vi "TouchPanel.ReadFKeys.vi"(7 "forced read (F)":bool, 8 "error in (no error)":errorcluster, 9 "Keyset to read":T1[](array[typedef]), 10 "key?":T1, 11 "mode (read key)":T2=enum."read key") -> (0 "error out":errorcluster, 2 "keyPressed":bool, 3 "Keyset out":T1[](array[typedef]))   [LabVIEW 2010]
uses:
  TouchPanel.keyMode.ctl
  TouchPanel.functionKeys.ctl
  LvSecure.dll
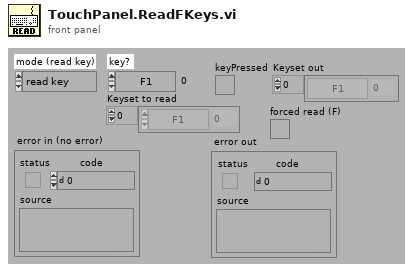
[diagram p1: front panel]
types:
  T1 = typedef "TouchPanel.functionKeys.ctl" = enum32{"F1", "F2", "F3", "F4", "F5", "F6", "F7", "F8", "F9", "F10", "F11", "F12", "Alt F1", "Alt F2", "Alt F3", "Alt F4", "Alt F5", "Alt F6", "Alt F7", "Alt F8", "Alt F9", "Alt F10", "Alt F11", "Alt F12", "Ctrl F1", "Ctrl F2", "Ctrl F3", "Ctrl F4", "Ctrl F5", "Ctrl F6", "Ctrl F7", "Ctrl F8", "Ctrl F9", "Ctrl F10", "Ctrl F11", "Ctrl F12", "Shift F1", "Shift F2", "Shift F3", "Shift F4", "Shift F5", "Shift F6", "Shift F7", "Shift F8", "Shift F9", "Shift F10", "Shift F11", "Shift F12", "Ctrl-Shift", "a", "b", "c", "d", "e", "f", "g", "h", "i", "j", "k", "l", "m", "n", "o", "p", "q", "r", "s", "t", "u", "v", "w", "x", "y", "z", "A", "B", "C", "D", "E", "F", "G", "H", "I", "J", "K", "L", "M", "N", "O", "P", "Q", "R", "S", "T", "U", "V", "W", "X", "Y", "Z", "0", "1", "2", "3", "4", "5", "6", "7", "8", "9", "Left", "Up", "Right", "Down", "Ctrl X", "Backspace", "Tab", "Enter", "Space", "End", "Home", "Insert", "Delete", ".", ","}
  T2 = typedef "TouchPanel.keyMode.ctl" = enum16{"init hook", "update keys", "read key", "read keyset", "read all", "simulate key", "mask keys", "unmask keys", "clear keys", "close hook"}
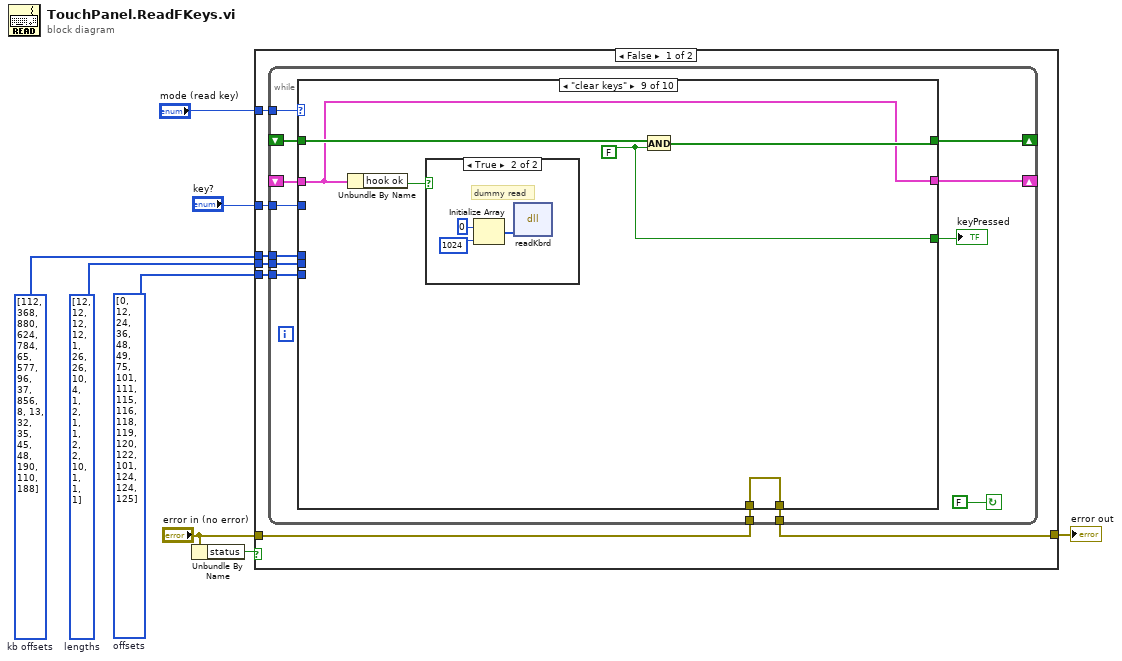
[diagram p0: block diagram]
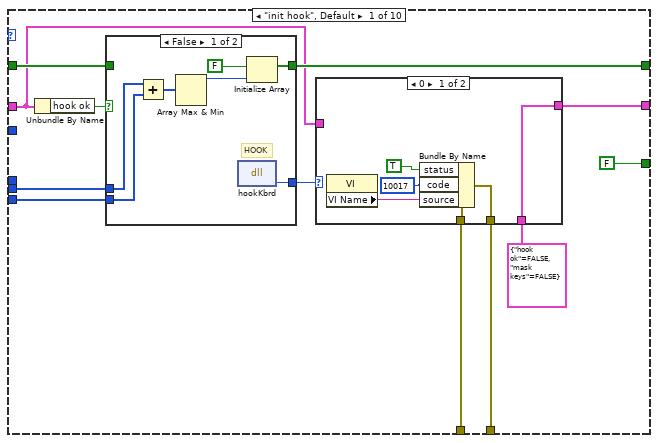
[diagram p2: hidden frame]
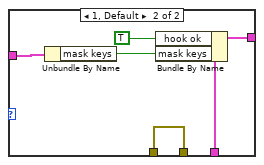
[diagram p3: hidden frame]
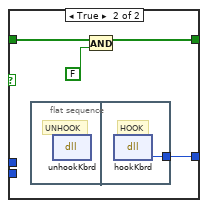
[diagram p4: hidden frame]
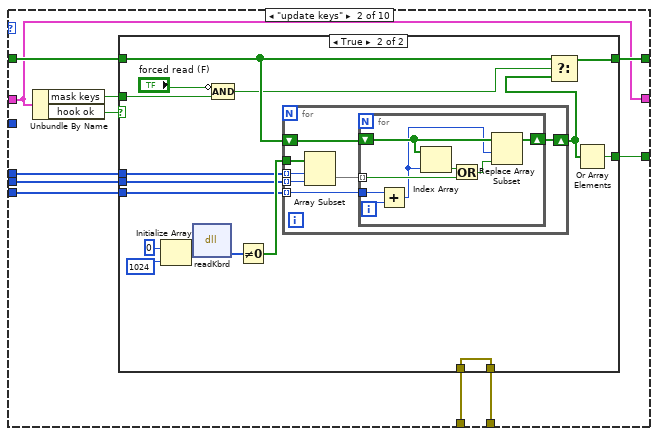
[diagram p5: hidden frame]
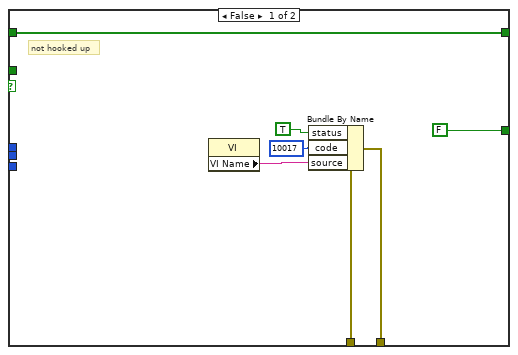
[diagram p6: hidden frame]
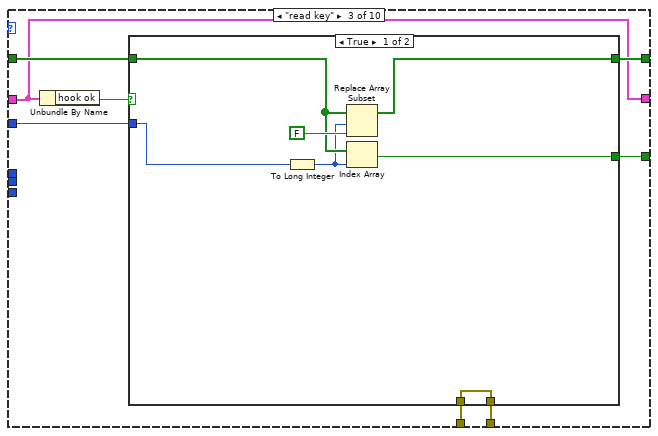
[diagram p7: hidden frame]
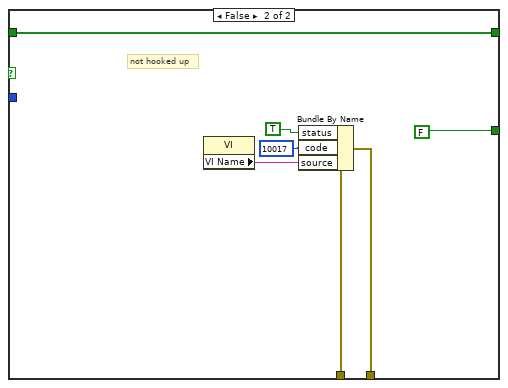
[diagram p8: hidden frame]
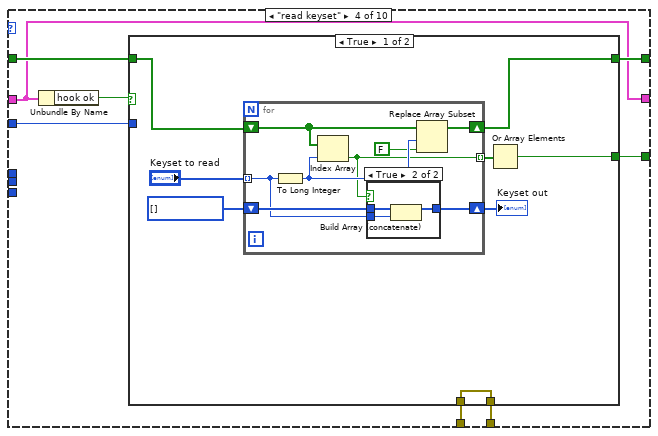
[diagram p9: hidden frame]
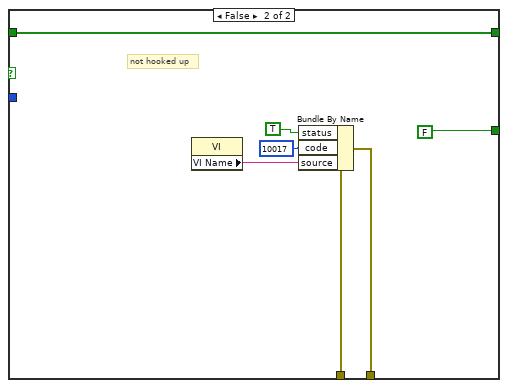
[diagram p11: hidden frame]
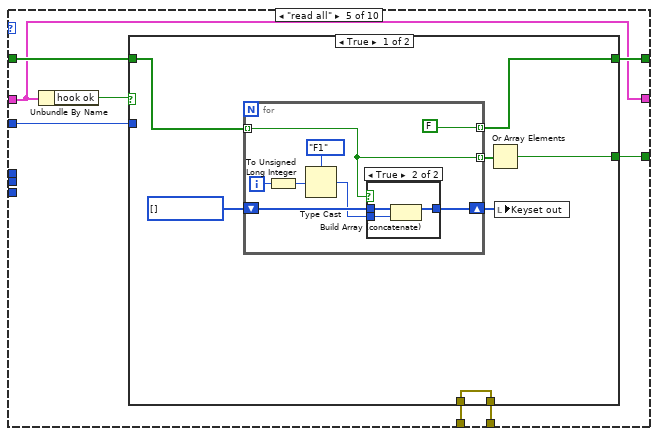
[diagram p12: hidden frame]
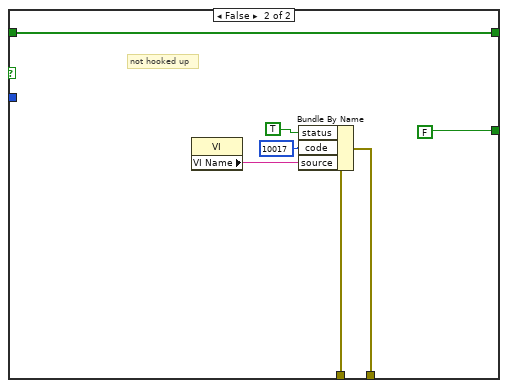
[diagram p14: hidden frame]
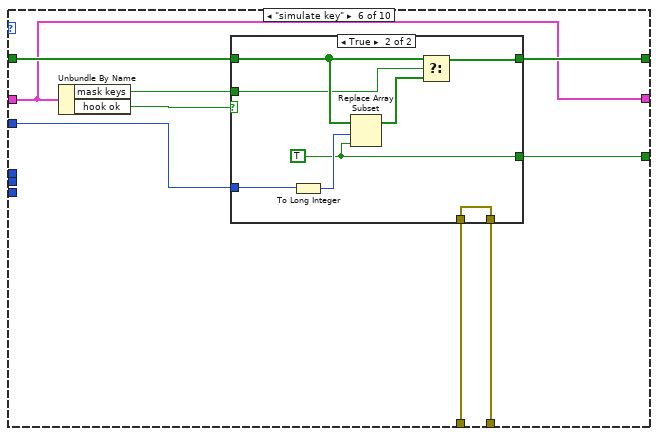
[diagram p15: hidden frame]
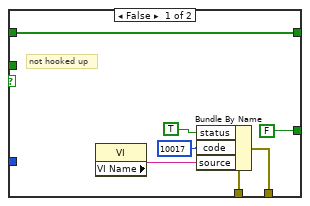
[diagram p16: hidden frame]
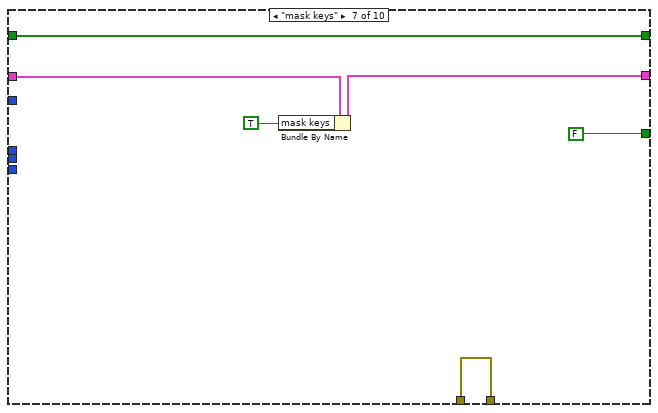
[diagram p17: hidden frame]
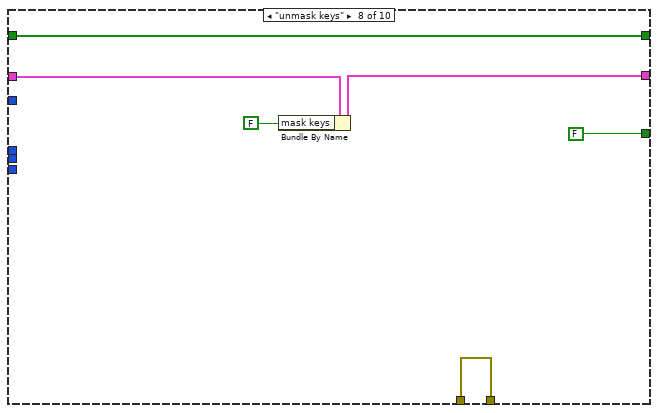
[diagram p18: hidden frame]
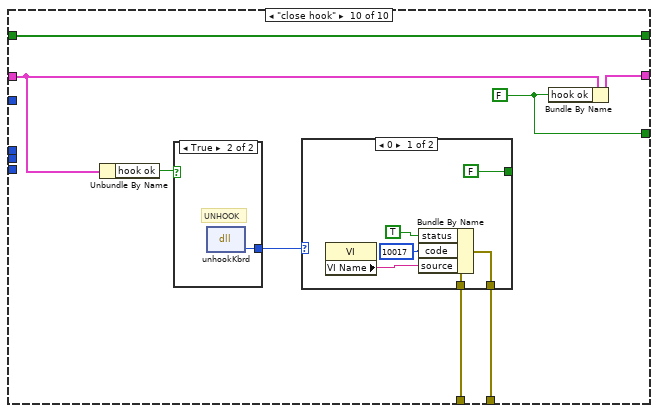
[diagram p20: hidden frame]
diagram:
  w1 = i32[] [0, 12, 24, 36, 48, 49, 75, 101, 111, 115, 116, 118, 119, 120, 122, 101, 124, 124, 125]  # offsets
  w2 = i32[] [12, 12, 12, 12, 1, 26, 26, 10, 4, 1, 2, 1, 1, 2, 2, 10, 1, 1, 1]  # lengths
  w3 = i32[] [112, 368, 880, 624, 784, 65, 577, 96, 37, 856, 8, 13, 32, 35, 45, 48, 190, 110, 188]  # kb offsets
  n1 = Unbundle By Name("error in (no error)") -> ("status"=w8:bool)
  n2 = case shown="False" w8 {
    tunnel: [w15 w268] -> w7
    tunnel: "error in (no error)" -> [w14 w268]
    tunnel: "mode (read key)" -> [w13 _]
    tunnel: "key?" -> [w12 _]
    tunnel: w3 -> [w11 _]
    tunnel: w2 -> [w10 _]
    tunnel: w1 -> [w9 _]
    frame False {
      n3 = while {
        tunnel: w9 -> [w18]
        tunnel: w10 -> [w19]
        tunnel: w11 -> [w20]
        tunnel: w12 -> [w22]
        shift-left: _ -> [w23]
        shift-right: [w17] -> _
        tunnel: w13 -> [w24]
        tunnel: [w25] -> w15
        tunnel: w14 -> [w26]
        shift-left: _ -> [w28]
        shift-right: [w27] -> _
        stop <- FALSE continue-if-true
        n4 = case shown="\"clear keys\"" w24 {
          tunnel: w28 -> [w29 w65 w114 w136 w171 w205 w232 w238 w242 w252]
          tunnel: [w37 w65 w114 w136 w171 w205 w231 w237 w242 w251] -> w27
          tunnel: w26 -> [w39 w74 w120 w142 w177 w212 w233 w239 w246 w256]
          tunnel: [w38 w75 w121 w143 w178 w213 w233 w239 w246 w255] -> w25
          tunnel: [w36 w73 w119 w141 w176 w211 w230 w236 w244 w254] -> w17
          tunnel: w23 -> [w35 w72 w118 w140 w175 w210 w230 w236 w245 w254]
          tunnel: w22 -> [_ _ w117 w139 w174 w209 _ _ _ _]
          tunnel: w20 -> [_ w71 _ _ _ _ _ _ _ _]
          tunnel: w19 -> [w34 w70 _ _ _ _ _ _ _ _]
          tunnel: w18 -> [w33 w69 _ _ _ _ _ _ _ _]
          tunnel: [FALSE ("Bundle Element") w68 w116 w138 w173 w208 FALSE ("Bundle Element") FALSE ("Bundle Element") w243 w250] -> w16
          frame "init hook", Default {
            n5 = Unbundle By Name(w29) -> ("hook ok"=w30:bool)
            n6 = case shown="False" w30 {
              tunnel: [w59 w63] -> w40
              tunnel: [w57 w61] -> w36
              tunnel: w35 -> [_ w62]
              tunnel: w34 -> [w56 _]
              tunnel: w33 -> [w55 _]
              frame False {
                # "HOOK"
                n7 = Add(x=w56, y=w55) -> (x+y=w53:i32[])
                n8 = Array Max & Min(array=w53) -> (max value=w54:i32)  [unwired: 3 out]
                n9 = dll-call lib="D:/work/PL_0246_Fiber_markup_validation/trunk/SOFTWARE/sources/tools/TouchPanel/LvSecure.dll" fn="hookKbrd"() -> (w59:i32)  [unwired: 3 in, 2 out]
                n10 = Initialize Array(FALSE ("Boolean"), w54) -> (w57:bool[])
              }
              frame True {
                n11 = flat-sequence {
                  tunnel: [w64] -> w63
                  frame #0 {
                    # "UNHOOK"
                    n12 = dll-call lib="D:/work/PL_0246_Fiber_markup_validation/trunk/SOFTWARE/sources/tools/TouchPanel/LvSecure.dll" fn="unhookKbrd"() -> ()  [unwired: 4 in, 2 out]
                  }
                  frame #1 {
                    # "HOOK"
                    n13 = dll-call lib="D:/work/PL_0246_Fiber_markup_validation/trunk/SOFTWARE/sources/tools/TouchPanel/LvSecure.dll" fn="hookKbrd"() -> (w64:i32)  [unwired: 3 in, 2 out]
                  }
                }
                n14 = And(x=w62, y=FALSE) -> (x .and. y?=w61:bool[])
              }
            }
            n15 = case shown="0" w40 {
              tunnel: [w42 w50] -> w37
              tunnel: w39 -> [w46 w52]
              tunnel: [w45 w52] -> w38
              tunnel: cluster{"hook ok":bool, "mask keys":bool} {"hook ok"=FALSE, "mask keys"=FALSE} -> [w42 w49]
              tunnel: w29 -> [_ w47]
              frame 0 {
                n16 = property class="VI"() -> ("VI Name"=w41:string)  [unwired: 2 in, 2 out]
                n17 = Bundle By Name(cluster=w46, "status"=TRUE ("Bundle Element"), "code"=10017 ("Bundle Element"), "source"=w41) -> (w45:errorcluster)
              }
              frame 1, Default {
                n18 = Unbundle By Name(w47) -> ("mask keys"=w48:bool)
                n19 = Bundle By Name(cluster=w49, "hook ok"=TRUE, "mask keys"=w48) -> (w50:cluster{"hook ok":bool, "mask keys":bool})
              }
            }
          }
          frame "update keys" {
            n20 = Unbundle By Name(w65) -> ("mask keys"=w66:bool, "hook ok"=w67:bool)
            n21 = case shown="True" w67 {
              tunnel: [w80 w98] -> w75
              tunnel: w74 -> [w79 w98]
              tunnel: [w78 w88] -> w73
              tunnel: w72 -> [w78 w89]
              tunnel: w71 -> [_ w92]
              tunnel: w70 -> [_ w91]
              tunnel: w69 -> [_ w90]
              tunnel: [FALSE ("Bundle Element") w86] -> w68
              tunnel: w66 -> [_ w85]
              frame False {
                # "not hooked up"
                n22 = property class="VI"() -> ("VI Name"=w76:string)  [unwired: 2 in, 2 out]
                n23 = Bundle By Name(cluster=w79, "status"=TRUE ("Bundle Element"), "code"=10017 ("Bundle Element"), "source"=w76) -> (w80:errorcluster)
              }
              frame True {
                n24 = Initialize Array(u8 0 ("Input Value"), 1024 ("Input Value")) -> (w96:u8[])
                n25 = dll-call lib="D:/work/PL_0246_Fiber_markup_validation/trunk/SOFTWARE/sources/tools/TouchPanel/LvSecure.dll" fn="readKbrd"("keyBoard"=w96) -> ("keyBoard"=w94:u8[])  [unwired: 4 in, 2 out]
                n26 = Compound Arithmetic op=AND(invert "forced read (F)", w85) -> (w83:bool)
                n27 = Not Equal To 0?(x=w94) -> (x != 0?=w97:bool[])
                n28 = for {
                  tunnel: w97 -> [w105]
                  shift-right: [w100] -> w87
                  shift-left: w89 -> [w102]
                  tunnel: w92 -> [w104] mode=indexing
                  tunnel: w91 -> [w103] mode=indexing
                  tunnel: w90 -> [w101] mode=indexing
                  n29 = Array Subset(array=w105, index=w104, length=w103) -> (w99:bool[])
                  n30 = for {
                    shift-right: [w110] -> w100
                    shift-left: w102 -> [w111]
                    tunnel: w101 -> [w113]
                    tunnel: w99 -> [w108] mode=indexing
                    i -> [w112]
                    n31 = Add(x=w113, y=w112) -> (x+y=w106:i32)
                    n32 = Index Array(array=w111, index=w106) -> (element=w109:bool)
                    n33 = Or(x=w109, y=w108) -> (x .or. y?=w107:bool)
                    n34 = Replace Array Subset(array=w111, new element=w107, index=w106) -> (w110:bool[])
                  }
                }
                n35 = Select(t=w89, s=w83, f=w87) -> (s? t:f=w88:bool[])
                n36 = Or Array Elements(Boolean array=w87) -> (logical OR=w86:bool)
              }
            }
          }
          frame "read key" {
            n37 = Unbundle By Name(w114) -> ("hook ok"=w115:bool)
            n38 = case shown="True" w115 {
              tunnel: [w128 w133] -> w121
              tunnel: w120 -> [w128 w132]
              tunnel: [w125 w131] -> w119
              tunnel: w118 -> [w126 w131]
              tunnel: w117 -> [w123 _]
              tunnel: [w122 FALSE ("Bundle Element")] -> w116
              frame True {
                n39 = To Long Integer(number=w123) -> (32bit integer=w124:i32)
                n40 = Replace Array Subset(array=w126, new element=FALSE ("Element Data"), index=w124) -> (w125:bool[])
                n41 = Index Array(array=w126, index=w124) -> (element=w122:bool)
              }
              frame False {
                # "not hooked up"
                n42 = property class="VI"() -> ("VI Name"=w129:string)  [unwired: 2 in, 2 out]
                n43 = Bundle By Name(cluster=w132, "status"=TRUE ("Bundle Element"), "code"=10017 ("Bundle Element"), "source"=w129) -> (w133:errorcluster)
              }
            }
          }
          frame "read keyset" {
            n44 = Unbundle By Name(w136) -> ("hook ok"=w137:bool)
            n45 = case shown="True" w137 {
              tunnel: [w151 w168] -> w143
              tunnel: w142 -> [w151 w167]
              tunnel: [w146 w166] -> w141
              tunnel: w140 -> [w147 w166]
              tunnel: w139 -> [_ _]
              tunnel: [w144 FALSE ("Bundle Element")] -> w138
              frame True {
                w150 = T1[] [] items=["F1", "F2", "F3", "F4", "F5", "F6", "F7", "F8", "F9", "F10", "F11", "F12", "Alt F1", "Alt F2", "Alt F3", "Alt F4", "Alt F5", "Alt F6", "Alt F7", "Alt F8", "Alt F9", "Alt F10", "Alt F11", "Alt F12", "Ctrl F1", "Ctrl F2", "Ctrl F3", "Ctrl F4", "Ctrl F5", "Ctrl F6", "Ctrl F7", "Ctrl F8", "Ctrl F9", "Ctrl F10", "Ctrl F11", "Ctrl F12", "Shift F1", "Shift F2", "Shift F3", "Shift F4", "Shift F5", "Shift F6", "Shift F7", "Shift F8", "Shift F9", "Shift F10", "Shift F11", "Shift F12", "Ctrl-Shift", "a", "b", "c", "d", "e", "f", "g", "h", "i", "j", "k", "l", "m", "n", "o", "p", "q", "r", "s", "t", "u", "v", "w", "x", "y", "z", "A", "B", "C", "D", "E", "F", "G", "H", "I", "J", "K", "L", "M", "N", "O", "P", "Q", "R", "S", "T", "U", "V", "W", "X", "Y", "Z", "0", "1", "2", "3", "4", "5", "6", "7", "8", "9", "Left", "Up", "Right", "Down", "Ctrl X", "Backspace", "Tab", "Enter", "Space", "End", "Home", "Insert", "Delete", ".", ","]
                n46 = for {
                  shift-right: [w153] -> w149
                  shift-left: w150 -> [w155]
                  tunnel: "Keyset to read" -> [w154] mode=indexing
                  shift-right: [w159] -> w146
                  shift-left: w147 -> [w158]
                  tunnel: [w152] -> w145 mode=indexing
                  n47 = To Long Integer(number=w154) -> (32bit integer=w157:i32)
                  n48 = Index Array(array=w158, index=w157) -> (element=w152:bool)
                  n49 = case shown="True" w152 {
                    tunnel: w155 -> [w160 w163]
                    tunnel: w154 -> [_ w162]
                    tunnel: [w160 w161] -> w153
                    frame False {
                    }
                    frame True {
                      n50 = Build Array (concatenate)(w163, w162) -> (w161:T1[])
                    }
                  }
                  n51 = Replace Array Subset(array=w158, new element=FALSE ("new element/subarray"), index=w157) -> (w159:bool[])
                }
                "Keyset out" <- w149
                n52 = Or Array Elements(Boolean array=w145) -> (logical OR=w144:bool)
              }
              frame False {
                # "not hooked up"
                n53 = property class="VI"() -> ("VI Name"=w164:string)  [unwired: 2 in, 2 out]
                n54 = Bundle By Name(cluster=w167, "status"=TRUE ("Bundle Element"), "code"=10017 ("Bundle Element"), "source"=w164) -> (w168:errorcluster)
              }
            }
          }
          frame "read all" {
            n55 = Unbundle By Name(w171) -> ("hook ok"=w172:bool)
            n56 = case shown="True" w172 {
              tunnel: [w185 w202] -> w178
              tunnel: w177 -> [w185 w201]
              tunnel: [w180 w200] -> w176
              tunnel: w175 -> [w181 w200]
              tunnel: w174 -> [_ _]
              tunnel: [w182 FALSE ("Bundle Element")] -> w173
              frame True {
                w184 = T1[] [] items=["F1", "F2", "F3", "F4", "F5", "F6", "F7", "F8", "F9", "F10", "F11", "F12", "Alt F1", "Alt F2", "Alt F3", "Alt F4", "Alt F5", "Alt F6", "Alt F7", "Alt F8", "Alt F9", "Alt F10", "Alt F11", "Alt F12", "Ctrl F1", "Ctrl F2", "Ctrl F3", "Ctrl F4", "Ctrl F5", "Ctrl F6", "Ctrl F7", "Ctrl F8", "Ctrl F9", "Ctrl F10", "Ctrl F11", "Ctrl F12", "Shift F1", "Shift F2", "Shift F3", "Shift F4", "Shift F5", "Shift F6", "Shift F7", "Shift F8", "Shift F9", "Shift F10", "Shift F11", "Shift F12", "Ctrl-Shift", "a", "b", "c", "d", "e", "f", "g", "h", "i", "j", "k", "l", "m", "n", "o", "p", "q", "r", "s", "t", "u", "v", "w", "x", "y", "z", "A", "B", "C", "D", "E", "F", "G", "H", "I", "J", "K", "L", "M", "N", "O", "P", "Q", "R", "S", "T", "U", "V", "W", "X", "Y", "Z", "0", "1", "2", "3", "4", "5", "6", "7", "8", "9", "Left", "Up", "Right", "Down", "Ctrl X", "Backspace", "Tab", "Enter", "Space", "End", "Home", "Insert", "Delete", ".", ","]
                n57 = for {
                  shift-right: [w192] -> w179
                  shift-left: w184 -> [w193]
                  tunnel: [w191] -> w183 mode=indexing
                  tunnel: w181 -> [w191] mode=indexing
                  tunnel: [FALSE ("new element/subarray")] -> w180 mode=indexing
                  i -> [w189]
                  n58 = To Unsigned Long Integer(number=w189) -> (unsigned 32bit integer=w187:u32)
                  n59 = Type Cast(type=TouchPanel.functionKeys."F1" ("key?"), x=w187) -> (*(type *) &x=w188:T1)
                  n60 = case shown="True" w191 {
                    tunnel: w193 -> [w194 w197]
                    tunnel: w188 -> [_ w196]
                    tunnel: [w194 w195] -> w192
                    frame False {
                    }
                    frame True {
                      n61 = Build Array (concatenate)(w197, w196) -> (w195:T1[])
                    }
                  }
                }
                n62 = Or Array Elements(Boolean array=w183) -> (logical OR=w182:bool)
                n63 = local write "Keyset out"(w179) -> ()
              }
              frame False {
                # "not hooked up"
                n64 = property class="VI"() -> ("VI Name"=w198:string)  [unwired: 2 in, 2 out]
                n65 = Bundle By Name(cluster=w201, "status"=TRUE ("Bundle Element"), "code"=10017 ("Bundle Element"), "source"=w198) -> (w202:errorcluster)
              }
            }
          }
          frame "simulate key" {
            n66 = Unbundle By Name(w205) -> ("mask keys"=w206:bool, "hook ok"=w207:bool)
            n67 = case shown="True" w207 {
              tunnel: [w218 w228] -> w213
              tunnel: w212 -> [w217 w228]
              tunnel: [w216 w223] -> w211
              tunnel: w210 -> [w216 w225]
              tunnel: w209 -> [_ w226]
              tunnel: [FALSE ("Bundle Element") w222] -> w208
              tunnel: w206 -> [_ w221]
              frame False {
                # "not hooked up"
                n68 = property class="VI"() -> ("VI Name"=w214:string)  [unwired: 2 in, 2 out]
                n69 = Bundle By Name(cluster=w217, "status"=TRUE ("Bundle Element"), "code"=10017 ("Bundle Element"), "source"=w214) -> (w218:errorcluster)
              }
              frame True {
                w222 = TRUE ("Element Data")
                n70 = To Long Integer(number=w226) -> (32bit integer=w227:i32)
                n71 = Replace Array Subset(array=w225, new element=w222, index=w227) -> (w224:bool[])
                n72 = Select(t=w225, s=w221, f=w224) -> (s? t:f=w223:bool[])
              }
            }
          }
          frame "mask keys" {
            n73 = Bundle By Name(cluster=w232, "mask keys"=TRUE) -> (w231:cluster{"hook ok":bool, "mask keys":bool})
          }
          frame "unmask keys" {
            n74 = Bundle By Name(cluster=w238, "mask keys"=FALSE) -> (w237:cluster{"hook ok":bool, "mask keys":bool})
          }
          frame "clear keys" {
            w243 = FALSE ("Succes")
            n75 = Unbundle By Name(w242) -> ("hook ok"=w241:bool)
            n76 = case shown="True" w241 {
              frame False {
              }
              frame True {
                # "dummy read"
                n77 = Initialize Array(u8 0 ("Input Value"), 1024 ("Input Value")) -> (w249:u8[])
                n78 = dll-call lib="D:/work/PL_0246_Fiber_markup_validation/trunk/SOFTWARE/sources/tools/TouchPanel/LvSecure.dll" fn="readKbrd"("keyBoard"=w249) -> ()  [unwired: 5 in, 2 out]
              }
            }
            n79 = And(x=w245, y=w243) -> (x .and. y?=w244:bool[])
          }
          frame "close hook" {
            w250 = FALSE
            n80 = Unbundle By Name(w252) -> ("hook ok"=w253:bool)
            n81 = case shown="True" w253 {
              tunnel: [w266 w267] -> w257
              frame False {
                w266 = 1  # not hooked up
              }
              frame True {
                # "UNHOOK"
                n82 = dll-call lib="D:/work/PL_0246_Fiber_markup_validation/trunk/SOFTWARE/sources/tools/TouchPanel/LvSecure.dll" fn="unhookKbrd"() -> (w267:i32)  [unwired: 3 in, 2 out]
              }
            }
            n83 = case shown="0" w257 {
              tunnel: [FALSE ("Succes") FALSE ("Succes")] -> _
              tunnel: w256 -> [w263 w265]
              tunnel: [w262 w265] -> w255
              frame 0 {
                n84 = property class="VI"() -> ("VI Name"=w258:string)  [unwired: 2 in, 2 out]
                n85 = Bundle By Name(cluster=w263, "status"=TRUE ("Bundle Element"), "code"=10017 ("Bundle Element"), "source"=w258) -> (w262:errorcluster)
              }
              frame 1, Default {
              }
            }
            n86 = Bundle By Name(cluster=w252, "hook ok"=w250) -> (w251:cluster{"hook ok":bool, "mask keys":bool})
          }
        }
        "keyPressed" <- w16
      }
    }
    frame True {
    }
  }
  "error out" <- w7
